vi "HWAsync Cmd Dialog.vi"(8 "error in (no error)":errorcluster) -> (0 "error out":errorcluster, 2 "Msg out":string)   [LabVIEW 2014]
panel:
  in  "Cluster":T1
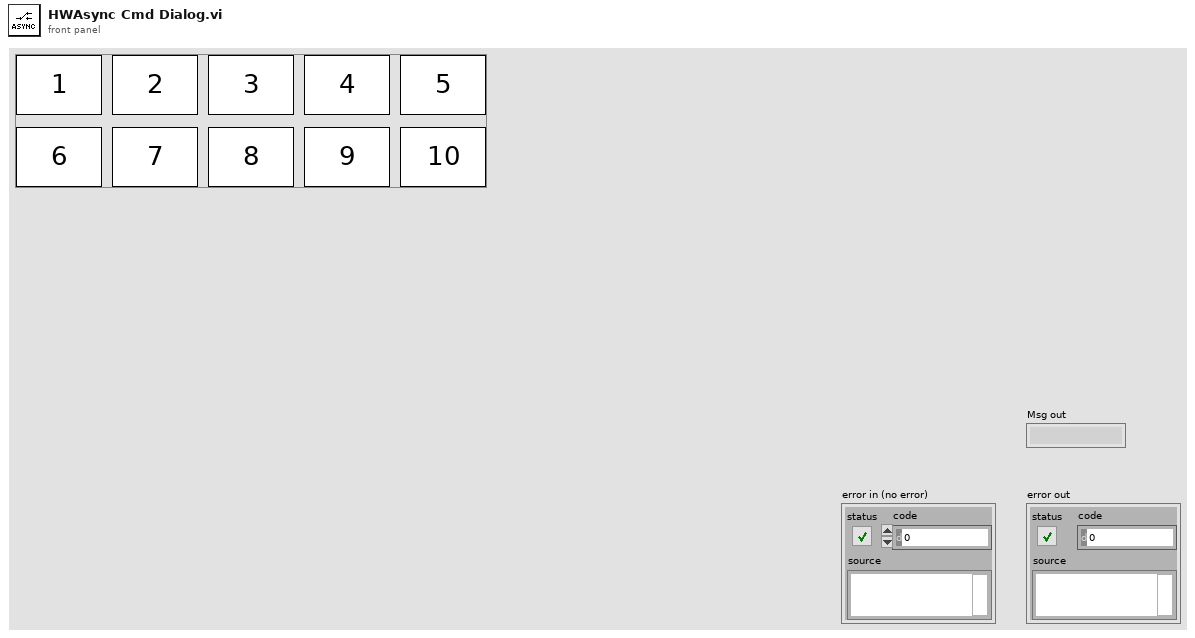
[diagram p1: front panel]
types:
  T1 = cluster{"HWSincrono 1":bool, "HWSincrono 2":bool, "HWSincrono 3":bool, "HWSincrono 4":bool, "HWSincrono 5":bool, "HWSincrono 6":bool, "HWSincrono 7":bool, "HWSincrono 8":bool, "HWSincrono 9":bool, "HWSincrono 10":bool}
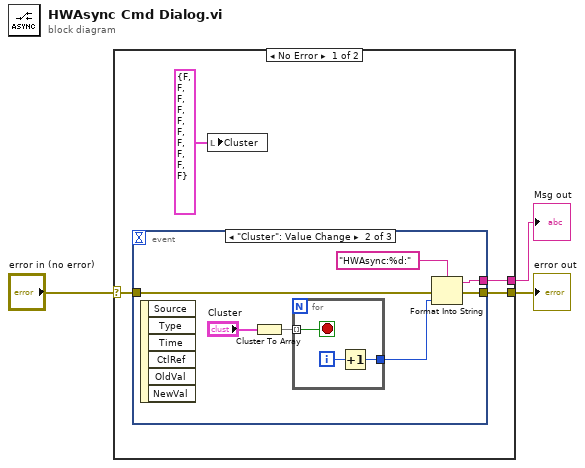
[diagram p0: block diagram]
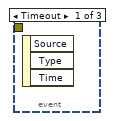
[diagram p2: hidden frame]
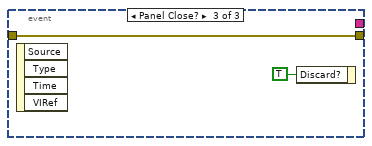
[diagram p3: hidden frame]
diagram:
  n1 = case shown="No Error" "error in (no error)" {
    selector: "error in (no error)" -> [w5 w20]
    tunnel: [w4 w20] -> w2
    tunnel: [w7 _] -> w1
    frame No Error {
      n2 = event shown="[1] \"Cluster\": Value Change" {
        selector: _ -> [_ _ _]
        dyn-events: _ -> [_ _ _]
        timeout: _ -> [_ _ _]
        tunnel: [_ w10 _] -> w7
        tunnel: w5 -> [_ w9 w18]
        tunnel: [_ w8 w18] -> w4
        event Timeout {
          n3 = event-data() -> ()  [unwired: 1 in, 3 out]
        }
        event "Cluster": Value Change {
          n4 = event-data() -> ()  [unwired: 1 in, 6 out]
          n5 = Cluster To Array(cluster="Cluster") -> (array=w13:bool[])
          n6 = for {
            tunnel: w13 -> [w17] mode=indexing
            tunnel: [w15] -> w11
            i -> [w16]
            stop <- w17 stop-if-true
            n7 = Increment(x=w16) -> (x+1=w15:i32)
          }
          n8 = Format Into String(format string="HWAsync:%d:", error in=w9, w11) -> (resulting string=w10:string, error out=w8:errorcluster)  [unwired: 1 in]
        }
        event Panel Close? {
          n9 = event-data() -> ()  [unwired: 1 in, 4 out]
          n10 = event-data("Discard?"=TRUE) -> ()  [unwired: 1 in, 1 out]
        }
      }
      n11 = local write "Cluster"(T1 {"HWSincrono 1"=FALSE, "HWSincrono 2"=FALSE, "HWSincrono 3"=FALSE, "HWSincrono 4"=FALSE, "HWSincrono 5"=FALSE, "HWSincrono 6"=FALSE, "HWSincrono 7"=FALSE, "HWSincrono 8"=FALSE, "HWSincrono 9"=FALSE, "HWSincrono 10"=FALSE} ("Cluster")) -> ()
    }
    frame Error {
    }
  }
  "Msg out" <- w1
  "error out" <- w2
